vi "Launch.vi"(8 "error in (no error)":errorcluster, 10 "Mediator":refnum<class "IMediator.lvclass">, 11 "MediatorBusMonitor in":refnum<class "MediatorBusMonitor.lvclass">) -> (0 "error out":errorcluster, 1 "Bus Monitor Enqueuer":refnum<class "Message Enqueuer.lvclass">, 2 "Mediator Out":refnum<class "IMediator.lvclass">)   [LabVIEW 2015, in "Mediator.lvlib" / "MediatorBusMonitor.lvclass"]
uses:
  MediatorBusMonitor.lvclass
  IMediator/IMediator/IMediator.lvclass
  <vilib>/ActorFramework/Message Enqueuer/Message Enqueuer.lvclass
  <vilib>/ActorFramework/Actor/Actor.lvclass
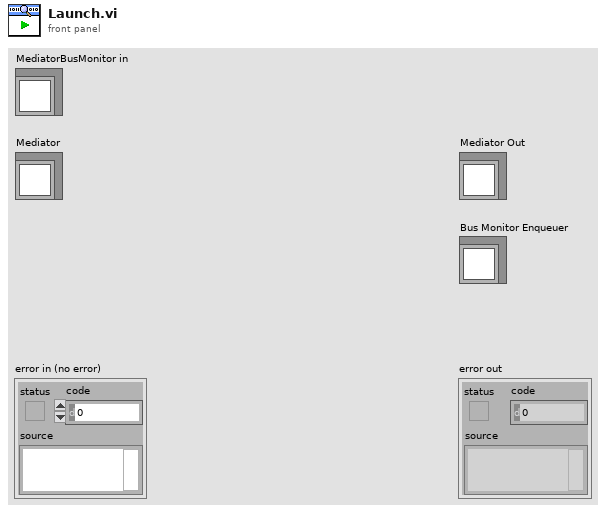
[diagram p1: front panel]
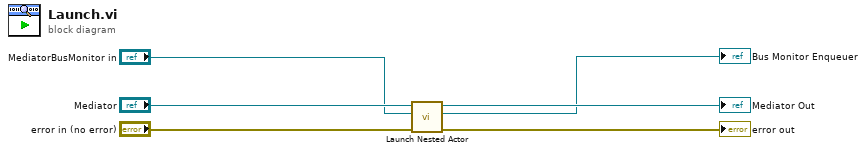
[diagram p0: block diagram]
diagram:
  n1 = call <vilib>:"Launch Nested Actor.vi"("error in (no error)"="error in (no error)", "Nested Actor"="MediatorBusMonitor in", "Caller Actor in"="Mediator") -> ("error out"=→"error out":errorcluster, "Nested Actor's Enqueuer"=→"Bus Monitor Enqueuer":refnum<class "Message Enqueuer.lvclass">, "Caller Actor out"=→"Mediator Out":refnum<class "IMediator.lvclass">)  [unwired: 6 in]
